vi "SetPosition_Choose2.vi"(0 "Choose2":refnum<vi>, 1 "FcdVI Refnum":refnum<vi>, 2 "Mode":refnum<vi>) -> ()   [LabVIEW 2014, in "Xgraph.xctl"]
uses:
  Xgraph.xctl
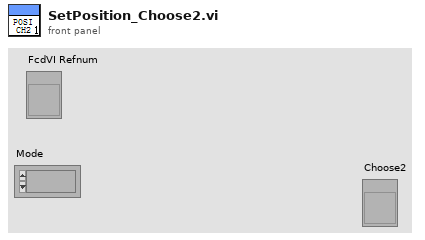
[diagram p1: front panel]
types:
  T1 = typedef "LVRectTypeDef.ctl" = cluster{"Left":i16, "Top":i16, "Right":i16, "Bottom":i16}
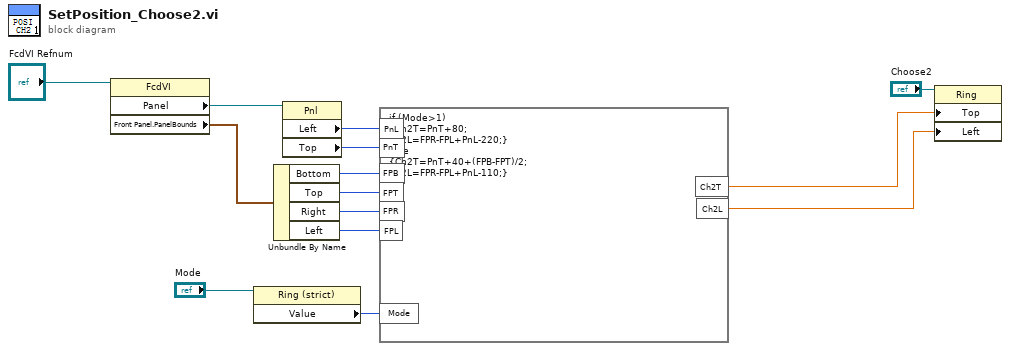
[diagram p0: block diagram]
diagram:
  n1 = property class="FcdVI"(reference="FcdVI Refnum") -> ("Panel"=w13:refnum<vi>, "Front Panel.PanelBounds"=w11:T1)  [unwired: 1 in, 2 out]
  n2 = property class="Ring (strict)"(reference="Mode") -> ("Value"=w1:u16)  [unwired: 1 in, 2 out]
  n3 = Unbundle By Name(w11) -> ("Bottom"=w10:i16, "Top"=w9:i16, "Right"=w8:i16, "Left"=w7:i16)
  n4 = property class="Pnl"(reference=w13) -> ("Left"=w3:i32, "Top"=w6:i32)  [unwired: 1 in, 2 out]
  n5 = formula code="if (Mode>1)\n{Ch2T=PnT+80;\nCh2L=FPR-FPL+PnL-220;}\nelse\n{Ch2T=PnT+40+(FPB-FPT)/2;\nCh2L=FPR-FPL+PnL-110;}"("FPB"=w10, "FPT"=w9, "FPR"=w8, "FPL"=w7, "PnT"=w6, "PnL"=w3, "Mode"=w1) -> ("Ch2T"=w5:dbl, "Ch2L"=w4:dbl)
  n6 = property class="Ring"(reference="Choose2", "Top"=w5, "Left"=w4) -> ()  [unwired: 1 in, 2 out]
